vi "broadcastFAForce.vi"(0 "ILCCommunications in":refnum<class "ILCCommunications.lvclass">, 5 "ModbusBuffer in":refnum<class "ModbusBuffer.lvclass">, 7 "Subnet":u8, 9 "SlewFlag":bool, 11 "error in (no error)":errorcluster) -> (4 "ILCCommunications out":refnum<class "ILCCommunications.lvclass">, 6 "ModbusBuffer out":refnum<class "ModbusBuffer.lvclass">, 15 "error out":errorcluster)   [LabVIEW 2016, in "ILCCommunications.lvclass"]
uses:
  ILCCommunications.lvclass
  Common_RT_Modbus/ModbusBuffer/ModbusBuffer.lvclass
  ILCCommunications.lvclass/ILCCommunications.ctl
  Common_RT_Modbus/ModbusBuffer/ModbusBuffer.lvclass/ModbusBuffer.ctl
  Common_RT_ILC/ILC/ILC.lvclass/ILC.ctl
  Common_RT_FAILC/FAILC/FAILC.lvclass/FAILC.ctl
  Common_RT_Modbus/ModbusBuffer/writeHeader.vi
  Common_RT_Modbus/ModbusBuffer/writeU8.vi
  Common_RT_FAILC/FAILC/determineSlewFlagValue.vi
  Common_RT_Modbus/ModbusBuffer/getIndex.vi
  Common_RT_Modbus/ModbusBuffer/setIndex.vi
  Common_RT_Modbus/ModbusBuffer/writeI24.vi
  Common_RT_Modbus/ModbusBuffer/writeCRC.vi
  Common_RT_Modbus/ModbusBuffer/writeDelay.vi
  Common_RT_Modbus/ModbusBuffer/writeEndOfFrame.vi
  Common_RT_Modbus/ModbusBuffer/writeByteInstruction.vi
  Common_RT_Modbus/ModbusBuffer/calculateCRC.vi
  Common_RT_FAILC/FAILC/FAILC.lvclass
  D:/Code/ts_M1M3Support/Common_RT_ILC/ILC/ILC.lvclass
  Common_RT_ILC/ILC/ILC.lvclass
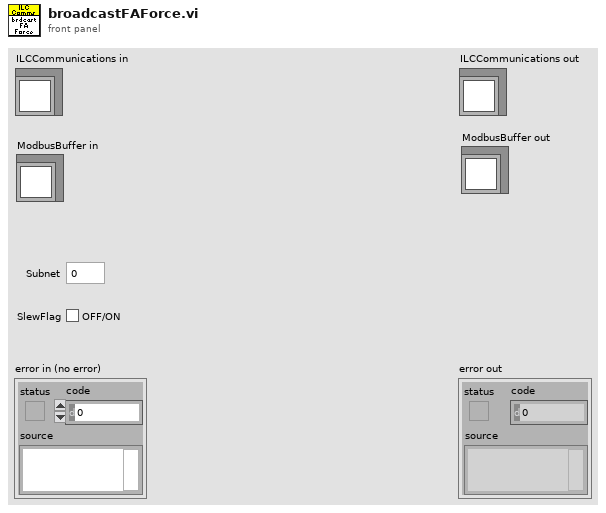
[diagram p1: front panel]
types:
  T1 = typedef "RTILC.lvlib/ILCData.ctl" = cluster{"Constants":T2, "Command":T3, "Telemetry":T5, "Responses":T6, "Timestamps":T8, "Timings":T9}
  T2 = typedef "RTILC.lvlib/ILCConstants.ctl" = cluster{"Subnet":u8, "Address":u8}
  T3 = typedef "RTILC.lvlib/ILCCommand.ctl" = cluster{"Mode":u16, "TemporaryAddress":u8, "ADCScanRate":T4, "ADCChannel":u8, "ADCOffset":sgl, "ADCSensitivity":sgl}
  T4 = typedef "RTILC.lvlib/ILCScanRates.ctl" = u8
  T5 = typedef "RTILC.lvlib/ILCTelemetry.ctl" = cluster{"UniqueID":u64, "FirmwareType":u8, "NetworkNodeType":u8, "ILCOption":u8, "NetworkNodeOption":u8, "MajorRevision":u8, "MinorRevision":u8, "FirmwareName":string, "Mode":u16, "MajorFault":bool, "MinorFault":bool, "FaultOverride":bool, "MainCalibrationError":bool, "BackupCalibrationError":bool, "UniqueIDCRCMismatch":bool, "AppTypeNodeTypeMismatch":bool, "AppMissing":bool, "AppCRCMismatch":bool, "TEDSNotFound":bool, "TEDS1Mismatch":bool, "TEDS2Mismatch":bool, "WatchdogResetDetected":bool, "BrownoutDetected":bool, "EventTrapResetDetected":bool, "MotorPowerFault":bool, "SSRPowerFault":bool, "AuxPowerFault":bool, "SMCPowerFault":bool, "TemporaryAddress":u8, "ADCScanRate":T4, "MainADCCalibrationK":sgl[], "MainSensorOffset":sgl[], "MainSensorSensitivity":sgl[], "BackupADCCalibrationK":sgl[], "BackupSensorOffset":sgl[], "BackupSensorSensitivity":sgl[]}
  T6 = typedef "RTILC.lvlib/ILCResponses.ctl" = cluster{"ReportServerID":T7, "ReportServerStatus":T7, "Mode":T7, "TemporaryAddress":T7, "Reset":T7, "ADCScanRate":T7, "ADCOffsetSensitivity":T7, "ReportCalibrationData":T7}
  T7 = typedef "RTModbus.lvlib/ExceptionCodes.ctl" = u16
  T8 = typedef "RTILC.lvlib/ILCTimestamps.ctl" = cluster{"ReportServerID":dbl, "ReportServerStatus":dbl, "Mode":dbl, "TemporaryAddress":dbl, "Reset":dbl, "ADCScanRate":dbl, "ADCOffsetSensitivity":dbl, "ReportCalibrationData":dbl}
  T9 = typedef "RTILC.lvlib/ILCTimings.ctl" = cluster{"ReportServerID":u32, "ReportServerStatus":u32, "Mode":u32, "TemporaryAddress":u32, "Reset":u32, "ADCScanRate":u32, "ADCOffsetSensitivity":u32, "ReportCalibrationData":u32}
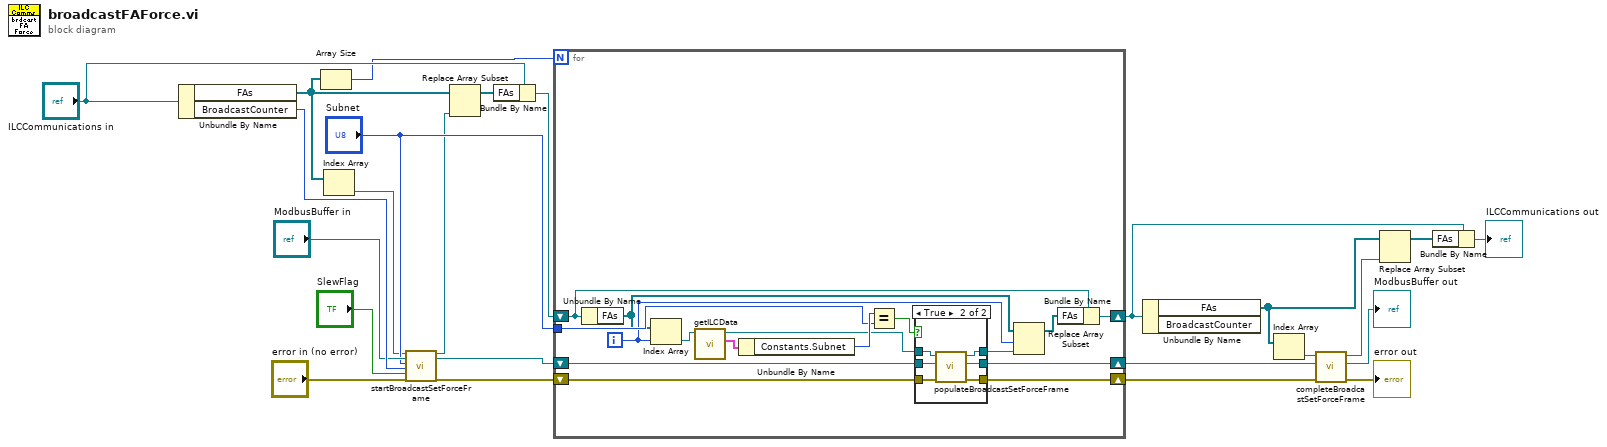
[diagram p0: block diagram]
diagram:
  n1 = Unbundle By Name("ILCCommunications in") -> ("FAs"=w2:refnum<class "FAILC.lvclass">[], "BroadcastCounter"=w24:u8)
  n2 = Array Size(array=w2) -> (size(s)=w1:i32)
  n3 = Index Array(array=w2) -> (element=w21:refnum<class "FAILC.lvclass">)  [unwired: 1 in]
  n4 = call "startBroadcastSetForceFrame.vi"("FAILC in"=w21, "ModbusBuffer in"="ModbusBuffer in", "Subnet"="Subnet", "BroadcastCounter"=w24, "SlewFlag"="SlewFlag", "error in (no error)"="error in (no error)") -> ("FAILC out"=w20:refnum<class "FAILC.lvclass">, "ModbusBuffer out"=w15:refnum<class "ModbusBuffer.lvclass">, "error out"=w6:errorcluster)  [unwired: 11 in]
  n5 = Replace Array Subset(array=w2, new element=w20) -> (w19:refnum<class "FAILC.lvclass">[])  [unwired: 1 in]
  n6 = Bundle By Name(cluster="ILCCommunications in", "FAs"=w19) -> (w17:refnum<class "ILCCommunications.lvclass">)
  n7 = for {
    N: w1 -> [_]
    shift-right: [w29] -> w8
    shift-left: w17 -> [w35]
    tunnel: "Subnet" -> [w37]
    shift-right: [w27] -> w11
    shift-left: w15 -> [w28]
    shift-right: [w26] -> w5
    shift-left: w6 -> [w25]
    i -> [w33]
    n8 = Unbundle By Name(w35) -> ("FAs"=w31:refnum<class "FAILC.lvclass">[])
    n9 = Index Array(array=w31, index=w33) -> (element=w40:refnum<class "FAILC.lvclass">)
    n10 = call "getILCData.vi"("ILC in"=w40) -> ("ILCData"=w39:T1, "ILC out"=w34:refnum<class "FAILC.lvclass">)  [unwired: 9 in]
    n11 = Unbundle By Name(w39) -> ("Constants.Subnet"=w38:u8)
    n12 = Equal?(x=w38, y=w37) -> (x = y?=w36:bool)
    n13 = case shown="True" w36 {
      tunnel: w34 -> [w43 w49]
      tunnel: [w43 w48] -> w32
      tunnel: w28 -> [w42 w47]
      tunnel: [w42 w46] -> w27
      tunnel: [w41 w44] -> w26
      tunnel: w25 -> [w41 w45]
      frame False {
      }
      frame True {
        n14 = call "populateBroadcastSetForceFrame.vi"("error in (no error)"=w45, "ModbusBuffer in"=w47, "FAILC in"=w49) -> ("error out"=w44:errorcluster, "ModbusBuffer out"=w46:refnum<class "ModbusBuffer.lvclass">, "FAILC out"=w48:refnum<class "FAILC.lvclass">)  [unwired: 6 in]
      }
    }
    n15 = Replace Array Subset(array=w31, new element=w32, index=w33) -> (w30:refnum<class "FAILC.lvclass">[])
    n16 = Bundle By Name(cluster=w35, "FAs"=w30) -> (w29:refnum<class "ILCCommunications.lvclass">)
  }
  n17 = Unbundle By Name(w8) -> ("FAs"=w14:refnum<class "FAILC.lvclass">[])  [unwired: 1 out]
  n18 = Index Array(array=w14) -> (element=w13:refnum<class "FAILC.lvclass">)  [unwired: 1 in]
  n19 = call "completeBroadcastSetForceFrame.vi"("error in (no error)"=w5, "ModbusBuffer in"=w11, "FAILC in"=w13) -> ("error out"=→"error out":errorcluster, "ModbusBuffer out"=→"ModbusBuffer out":refnum<class "ModbusBuffer.lvclass">, "FAILC out"=w12:refnum<class "FAILC.lvclass">)  [unwired: 6 in]
  n20 = Replace Array Subset(array=w14, new element=w12) -> (w9:refnum<class "FAILC.lvclass">[])  [unwired: 1 in]
  n21 = Bundle By Name(cluster=w8, "FAs"=w9) -> (→"ILCCommunications out":refnum<class "ILCCommunications.lvclass">)
